vi "AutoLauncher.vi"(11 "# Frisbees":i32) -> ()   [LabVIEW 2012]
uses:
  State_Machine_Enum.ctl
  Robot Global Data.vi
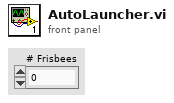
[diagram p1: front panel]
types:
  T1 = typedef "State_Machine_Enum.ctl" = enum16{"Idle", "Start", "Do", "Stop", "Init"}
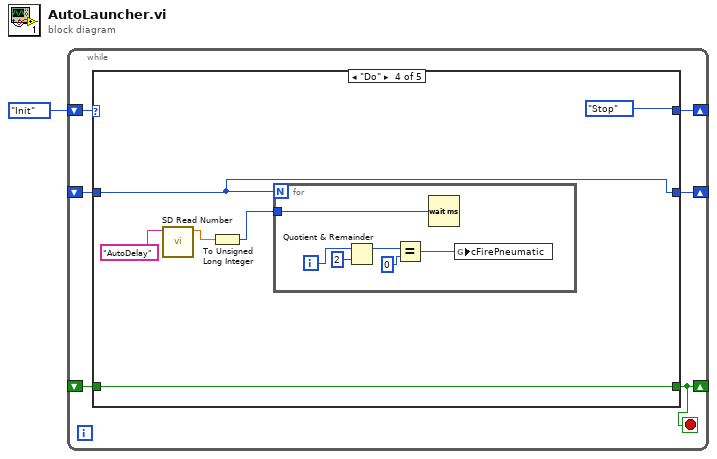
[diagram p0: block diagram]
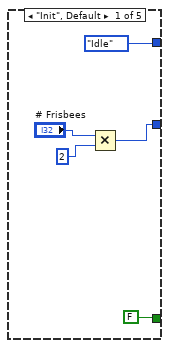
[diagram p2: hidden frame]
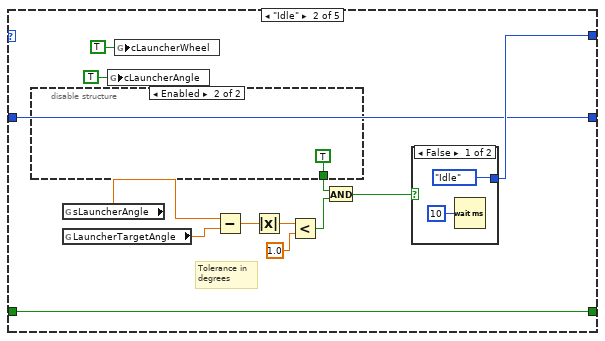
[diagram p3: hidden frame]
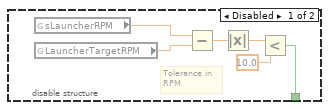
[diagram p4: hidden frame]
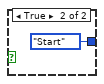
[diagram p5: hidden frame]
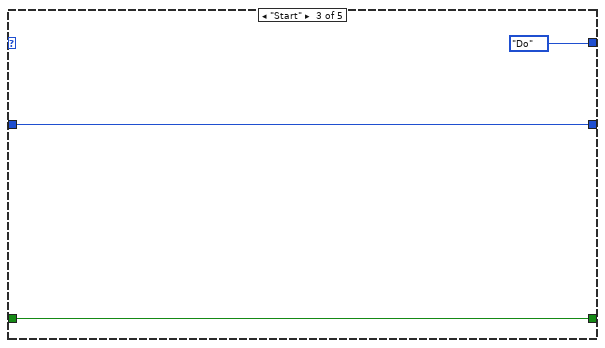
[diagram p6: hidden frame]
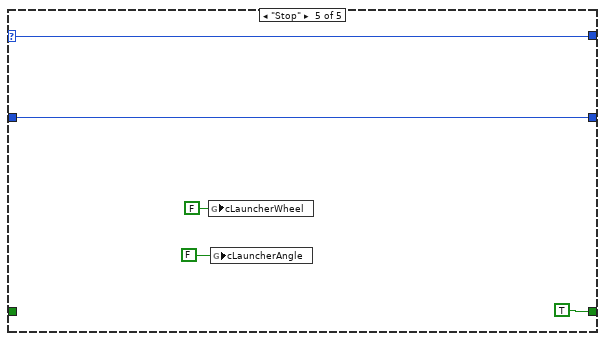
[diagram p7: hidden frame]
diagram:
  n1 = while {
    shift-right: [w6] -> _
    shift-left: State_Machine_Enum."Init" ("State") -> [w7]
    shift-right: [w5] -> _
    shift-left: _ -> [w4]
    shift-right: [w3] -> _
    shift-left: _ -> [w2]
    stop <- w5 stop-if-true
    n2 = case shown="\"Do\"" w7 {
      selector: w7 -> [_ _ _ _ w53]
      tunnel: [State_Machine_Enum."Idle" ("State") w16 State_Machine_Enum."Do" ("State") State_Machine_Enum."Stop" ("State") w53] -> w6
      tunnel: [FALSE w25 w37 w43 TRUE] -> w5
      tunnel: w4 -> [_ w25 w37 w43 _]
      tunnel: [w8 w15 w36 w44 w54] -> w3
      tunnel: w2 -> [_ w15 w36 w44 w54]
      frame "Init", Default {
        n3 = Multiply(x="# Frisbees", y=2) -> (x*y=w8:i32)
      }
      frame "Idle" {
        # "Tolerance in\ndegrees"
        n4 = disable-structure shown="Enabled" {
          disable-tunnel: [w26 TRUE] -> w18
          frame Disabled {
            # "Tolerance in\nRPM"
            n5 = global read "Robot Global Data.vi" "sLauncherRPM"() -> (w31:dbl)
            n6 = global read "Robot Global Data.vi" "LauncherTargetRPM"() -> (w30:dbl)
            n7 = Subtract(x=w31, y=w30) -> (x-y=w29:dbl)
            n8 = Absolute Value(x=w29) -> (abs(x)=w28:dbl)
            n9 = Less?(x=w28, y=10.0) -> (x < y?=w26:bool)
          }
          frame Enabled {
          }
        }
        n10 = global read "Robot Global Data.vi" "sLauncherAngle"() -> (w24:dbl)
        n11 = global read "Robot Global Data.vi" "LauncherTargetAngle"() -> (w23:dbl)
        n12 = global write "Robot Global Data.vi" "cLauncherAngle"(TRUE ("cLauncherAngle")) -> ()
        n13 = global write "Robot Global Data.vi" "cLauncherWheel"(TRUE ("cLauncherWheel")) -> ()
        n14 = Subtract(x=w24, y=w23) -> (x-y=w22:dbl)
        n15 = Absolute Value(x=w22) -> (abs(x)=w21:dbl)
        n16 = Less?(x=w21, y=1.0) -> (x < y?=w19:bool)
        n17 = And(x=w18, y=w19) -> (x .and. y?=w17:bool)
        n18 = case shown="False" w17 {
          tunnel: [State_Machine_Enum."Idle" ("State") State_Machine_Enum."Start" ("State")] -> w16
          frame False {
            n19 = Wait (ms)(milliseconds to wait=u32 10) -> ()  [unwired: 1 out]
          }
          frame True {
          }
        }
      }
      frame "Start" {
      }
      frame "Do" {
        n20 = call <vilib>:"SD Read Number.vi"("Name"="AutoDelay") -> ("Numeric"=w40:dbl)  [unwired: 8 in, 2 out]
        n21 = To Unsigned Long Integer(number=w40) -> (unsigned 32bit integer=w39:u32)
        n22 = for {
          N: w44 -> [_]
          tunnel: w39 -> [w45]
          i -> [w50]
          n23 = Quotient & Remainder(x=w50, y=2) -> (x-y*floor(x/y)=w48:i32)  [unwired: 1 out]
          n24 = Equal?(x=w48, y=0) -> (x = y?=w46:bool)
          n25 = Wait (ms)(milliseconds to wait=w45) -> ()  [unwired: 1 out]
          n26 = global write "Robot Global Data.vi" "cFirePneumatic"(w46) -> ()
        }
      }
      frame "Stop" {
        n27 = global write "Robot Global Data.vi" "cLauncherWheel"(FALSE ("cLauncherWheel")) -> ()
        n28 = global write "Robot Global Data.vi" "cLauncherAngle"(FALSE ("cLauncherWheel")) -> ()
      }
    }
  }
